vi "Format Metadata.vi"(0 "Waveform in":refnum<class "Waveform.lvclass">, 7 "Prefix":string, 11 "error in (no error)":errorcluster) -> (4 "Waveform out":refnum<class "Waveform.lvclass">, 8 "String":string, 15 "error out":errorcluster)   [LabVIEW 2015, in "Waveform.lvclass"]
uses:
  Waveform.lvclass
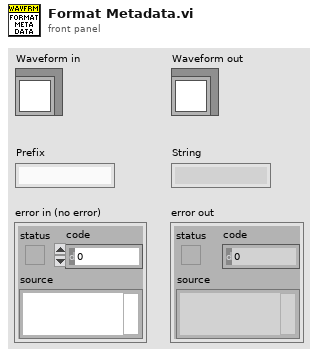
[diagram p1: front panel]
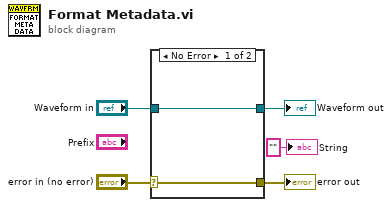
[diagram p0: block diagram]
diagram:
  n1 = case shown="No Error" "error in (no error)" {
    selector: "error in (no error)" -> [w6 w9]
    tunnel: [w6 w9] -> w4
    tunnel: [w7 w8] -> w2
    tunnel: "Waveform in" -> [w7 w8]
    frame No Error {
    }
    frame Error {
    }
  }
  "error out" <- w4
  "Waveform out" <- w2
  "String" <- "" ("String")
